vi "demo - tunnel while loop.vi"() -> ()   [LabVIEW 2024]
doc: "#vi_description \nPlot a sine wave onto a waveform chart with user adjustable wavelength\nThetic Engineering Ltd."
panel:
  in  "Wavelength":u8(slide)=6 min=1 scale=1.0..10.0
  in  "Stop":bool
  out "Waveform Chart":dbl(graph)
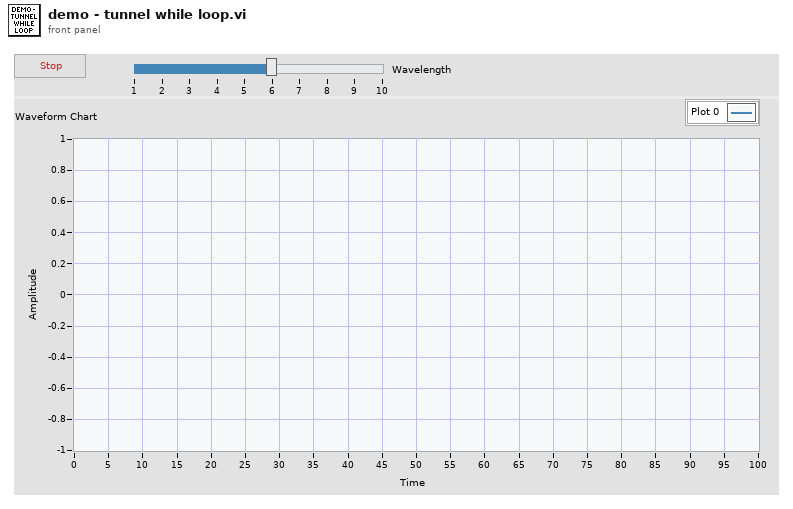
[diagram p1: front panel]
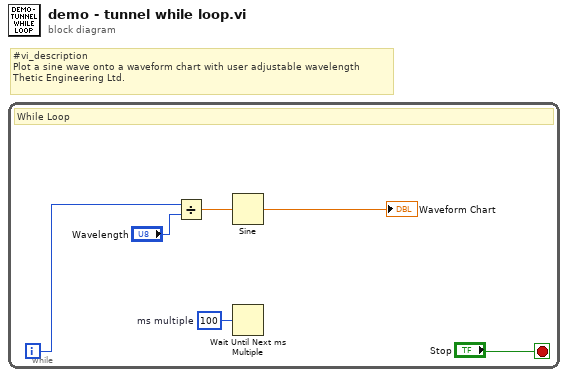
[diagram p0: block diagram]
diagram:
  # "#vi_description \nPlot a sine wave onto a waveform chart with user adjustable wavelength\nThetic Engineering Ltd."
  n1 = while {
    i -> [w4]
    stop <- "Stop" stop-if-true
    w2 = u32 100  # ms multiple
    # "While Loop"
    n2 = Divide(x=w4, y="Wavelength") -> (x/y=w3:dbl)
    n3 = Sine(x=w3) -> (sin(x)=→"Waveform Chart":dbl)
    n4 = Wait Until Next ms Multiple(millisecond multiple=w2) -> ()  [unwired: 1 out]
  }
